vi "Resolve Startup Promise.vi"(8 "error in (no error)":errorcluster, 11 "VolatusCore in":refnum<class "VolatusCore.lvclass">) -> (0 "error out":errorcluster, 3 "VolatusCore out":refnum<class "VolatusCore.lvclass">)   [LabVIEW 2020, in "Volatus.lvlib" / "VolatusCore.lvclass"]
uses:
  VolatusCore.lvclass
  VolatusCore.lvclass/VolatusCore.ctl
  AppStartupValue/AppStartupValue.lvclass/AppStartupValue.ctl
  AppStartupValue/AppStartupValue.lvclass
  C:/dev/lv20CE/relink/lv-promises/Promises/Value/Value.lvclass
  lv-promises/Promises/Promise/Promise.lvclass
  Event API/EventAPI.lvclass
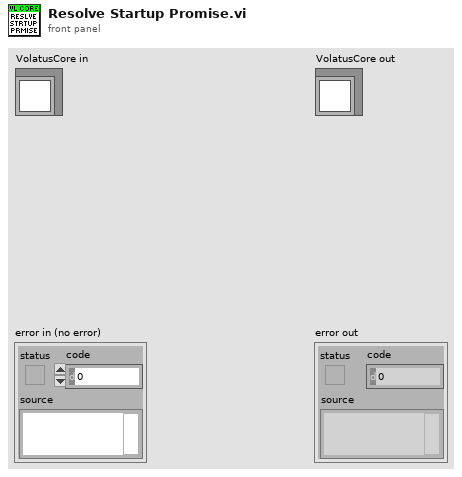
[diagram p1: front panel]
types:
  T1 = typedef "Volatus.lvlib/Event.ctl" = cluster{"Level":T2, "Context":string, "Message":string, "Error":errorcluster, "Time Stamp":timestamp}
  T2 = typedef "Volatus.lvlib/Event Level.ctl" = enum16{"Debug", "Info", "Warning", "Error"}
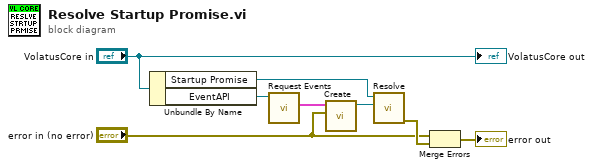
[diagram p0: block diagram]
diagram:
  n1 = Unbundle By Name("VolatusCore in") -> ("Startup Promise"=w8:refnum<class "Promise.lvclass">, "EventAPI"=w4:refnum<class "EventAPI.lvclass">)
  n2 = call "Request Events.vi"("EventAPI in"=w4) -> ("Events"=w3:T1[])  [unwired: 8 in, 2 out]
  n3 = call "Create.vi"("error in (no error)"="error in (no error)", "Events"=w3) -> ("AppStartupValue out"=w1:refnum<class "AppStartupValue.lvclass">)  [unwired: 8 in, 1 out]
  n4 = call "Resolve.vi"("Result"=w1, "Promise in"=w8) -> ("error out"=w6:errorcluster)  [unwired: 8 in, 1 out]
  n5 = Merge Errors("error in (no error)", w6) -> (→"error out":errorcluster)
  "VolatusCore out" <- "VolatusCore in"
